vi "PID_RT.vi"() -> ()   [LabVIEW 2017]
uses:
  <vilib>/myRIO/Instrument Drivers/Onboard IO/AO/typedefs/AO Reference.ctl
  <vilib>/myRIO/Common/Instrument Driver Framework/Utilities/typedefs/myRIO Generic Hardware Reference.ctl
  <vilib>/myRIO/Common/Instrument Driver Framework/Utilities/typedefs/Hardware Version Enum.ctl
  <vilib>/myRIO/Common/Instrument Driver Framework/Utilities/typedefs/myRIO v1.0 Reference.ctl
  <vilib>/myRIO/Common/Instrument Driver Framework/Utilities/typedefs/Generic FPGA Reference.ctl
  <vilib>/myRIO/Common/Instrument Driver Framework/myRIO v1.0/AO/typedefs/AO Channels List.ctl
  <vilib>/myRIO/Common/Instrument Driver Framework/myRIO v1.0/AO/typedefs/AO Channels Enum.ctl
  <vilib>/myRIO/Common/Instrument Driver Framework/Utilities/typedefs/Analog Scaling Constants List.ctl
  <vilib>/myRIO/Common/Instrument Driver Framework/Utilities/typedefs/Analog Scaling Constants.ctl
  <vilib>/userdefined/High Color/nirio_resource_hc.ctl
  <vilib>/Platform/TimedLoop/XDataNode/timing_clust.ctl
  <vilib>/Platform/TimedLoop/XDataNode/nitl_modes.ctl
  <vilib>/Platform/TimedLoop/XDataNode/wakeup.ctl
  <vilib>/myRIO/Common/Instrument Driver Framework/Utilities/vis/Is FPGA Ref Available.vi
  <vilib>/myRIO/Common/Instrument Driver Framework/myRIO v1.0/AO/vis/myRIO v1.1 Open AO.vi
  <vilib>/myRIO/Instrument Drivers/Onboard IO/AO/vis/Write.vi
  <vilib>/myRIO/Common/Instrument Driver Framework/Utilities/vis/Validate Channels.vi
  <vilib>/myRIO/Common/Instrument Driver Framework/myRIO v1.0/AO/vis/myRIO v1.0 Reserve AO.vi
  <vilib>/myRIO/Common/Instrument Driver Framework/myRIO v1.0/AO/vis/myRIO v1.0 Build MUX Configuration AO.vi
  <vilib>/myRIO/Common/Instrument Driver Framework/myRIO v1.0/Resource Manager/vis/myRIO v1.0 Reserve Channel List.vi
  <vilib>/myRIO/Common/Instrument Driver Framework/myRIO v1.0/Resource Manager/vis/myRIO v1.0 Reserve Channel.vi
  <vilib>/myRIO/Common/Instrument Driver Framework/myRIO v1.0/Resource Manager/vis/myRIO v1.0 Unreserve Channel.vi
  <vilib>/myRIO/Common/Instrument Driver Framework/myRIO v1.0/Resource Manager/vis/myRIO v1.0 Build Mutex Name.vi
  <vilib>/Utility/VariantDataType/GetNumericInfo.vi
  <vilib>/Utility/error.llb/Error Cluster From Error Code.vi
  <vilib>/myRIO/Common/Instrument Driver Framework/myRIO v1.0/myRIO v1.1 Open.vi
  <vilib>/myRIO/Common/Instrument Driver Framework/myRIO v1.0/AO/vis/myRIO v1.0 Get Scaling Constants AO.vi
  <vilib>/myRIO/Common/Instrument Driver Framework/Utilities/vis/IO Manager.vi
  <vilib>/myRIO/Common/Instrument Driver Framework/Utilities/vis/Configuration Manager.vi
  <vilib>/myRIO/Common/Instrument Driver Framework/myRIO v1.0/myRIO v1.0 Close.vi
  <vilib>/myRIO/Common/Instrument Driver Framework/myRIO v1.0/AO/vis/myRIO v1.0 Write AO.vi
  <vilib>/addons/control/pid/pid.llb/PID (DBL).vi
  <vilib>/myRIO/Express VI/Onboard IO/AO/AO Express VI.xnode
  <vilib>/myRIO/Instrument Drivers/Onboard IO/AO/vis/myRIO AO Open.xnode
  <vilib>/platform/TimedLoop/XDataNode/XDataNode.xnode
  <vilib>/addons/control/pid/NI_PID_pid.lvlib
  <vilib>/myRIO/Instrument Drivers/Onboard IO/AO/AO.lvlib
  <vilib>/Platform/TimedLoop/XDataNode/XDNodeRunTimeDep.lvlib
panel:
  out "Yel":bool
  out "Red":bool
  out "Grn":bool
  out "Speeding Up?":bool
  out "Velocity":dbl(graph)
  in  "stop":bool
  out "error out":errorcluster
  out "process variable":dbl
  out "Setpoint":dbl
  out "Analog Output":dbl(graph)=3.193359702
  out "output":dbl format="%.2f"
  out "Theta":cluster{"setpoint":dbl, dbl}(graph)={"setpoint"=303.908879655711, 0.0}
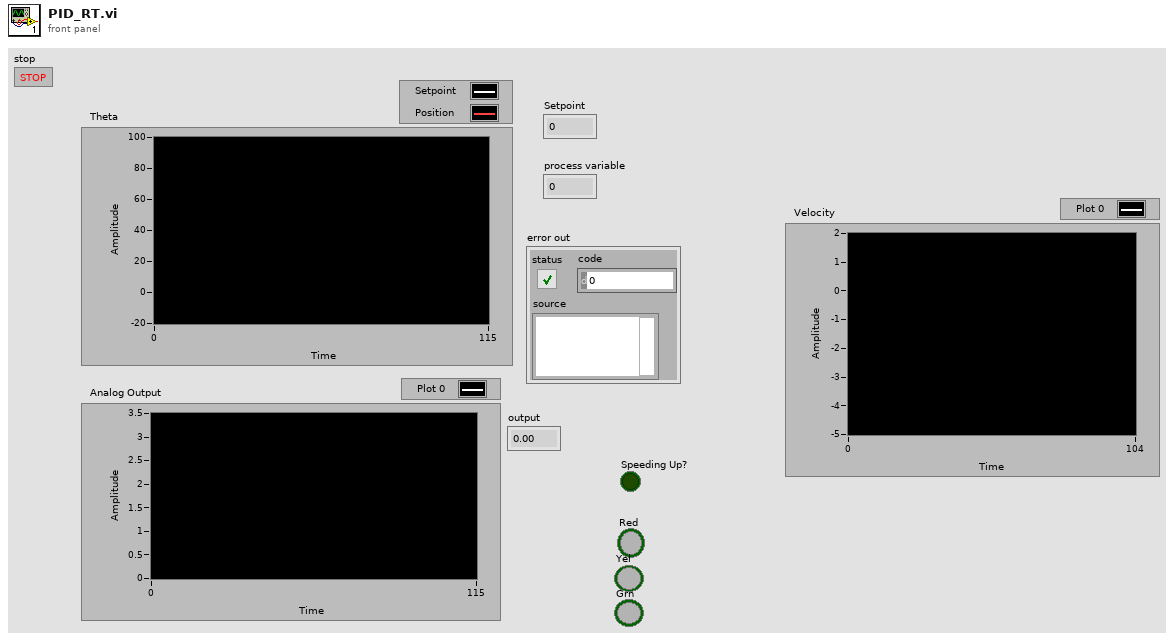
[diagram p1: front panel]
types:
  T1 = typedef "AO.lvlib/AO Reference.ctl" = cluster{"myRIO Reference":T2, "AO Channel List":T6, "AO Scaling Constant List":T8}
  T2 = typedef "myRIO Generic Hardware Reference.ctl" = cluster{"myRIO Model":T3, "myRIO Hardware Reference":T4}
  T3 = typedef "Hardware Version Enum.ctl" = enum16{"Unknown", "myRIO-1900", "myRIO-1950", "roboRIO", "NI ELVIS RIO CM"}
  T4 = typedef "myRIO v1.0 Reference.ctl" = cluster{"Generic FPGA Reference":T5, "Allow multiple opens":bool}
  T5 = typedef "Generic FPGA Reference.ctl" = refnum<k20>
  T6 = typedef "AO Channels List.ctl" = T7[]
  T7 = typedef "AO Channels Enum.ctl" = enum16{"Not Connected", "AudioOut/Left", "AudioOut/Right", "C/AO0", "C/AO1", "A/AO0", "A/AO1", "B/AO0", "B/AO1"}
  T8 = typedef "Analog Scaling Constants List.ctl" = T9[]
  T9 = typedef "Analog Scaling Constants.ctl" = cluster{"LSB Weight (Volts)":dbl, "Offset (Volts)":dbl, "Signed?":bool}
  T10 = typedef "nirio_resource_hc.ctl" = tag
  T11 = typedef "XDNodeRunTimeDep.lvlib/timing_clust.ctl" = cluster{"Expected End [f-1]":u64, "Actual End [f-1]":u64, "Finished Late? [f-1]":bool, "Expected End [i-1]":u64, "Actual End [i-1]":u64, "Finished Late? [i-1]":bool, "Expected Start [i]":u64, "Actual Start [i]":u64, "Expected Start [f]":u64, "Actual Start [f]":u64, "Source Name":string, "Structure Name":string, "Period":i64, "Deadline":i64, "Offset":i64, "Start":i64, "Priority":i32, "Timeout":i32, "Mode":T12, "Wakeup Reason":T13, "Error":errorcluster, "Source Type":string, "Secondary Source Type":string, "Global End Time":u64, "Global Start Time":u64, "Frame Duration":u64, "Iteration Duration":u64, "Assigned CPU":i32, "I/O Scan Engine Mode":u32}
  T12 = typedef "XDNodeRunTimeDep.lvlib/nitl_modes.ctl" = enum32{"No Change", "Process missed periods, maintain original phase", "Discard missed periods, maintain original phase", "Process missed periods, ignore original phase", "Discard missed periods, ignore original phase"}
  T13 = typedef "XDNodeRunTimeDep.lvlib/wakeup.ctl" = enum32{"Normal", "Aborted", "Asynchronous wakeup", "Timing source error", "Timed loop error", "Timeout"}
  T14 = cluster{"proportional gain (Kc)":dbl, "integral time (Ti, min)":dbl, "derivative time (Td, min)":dbl}
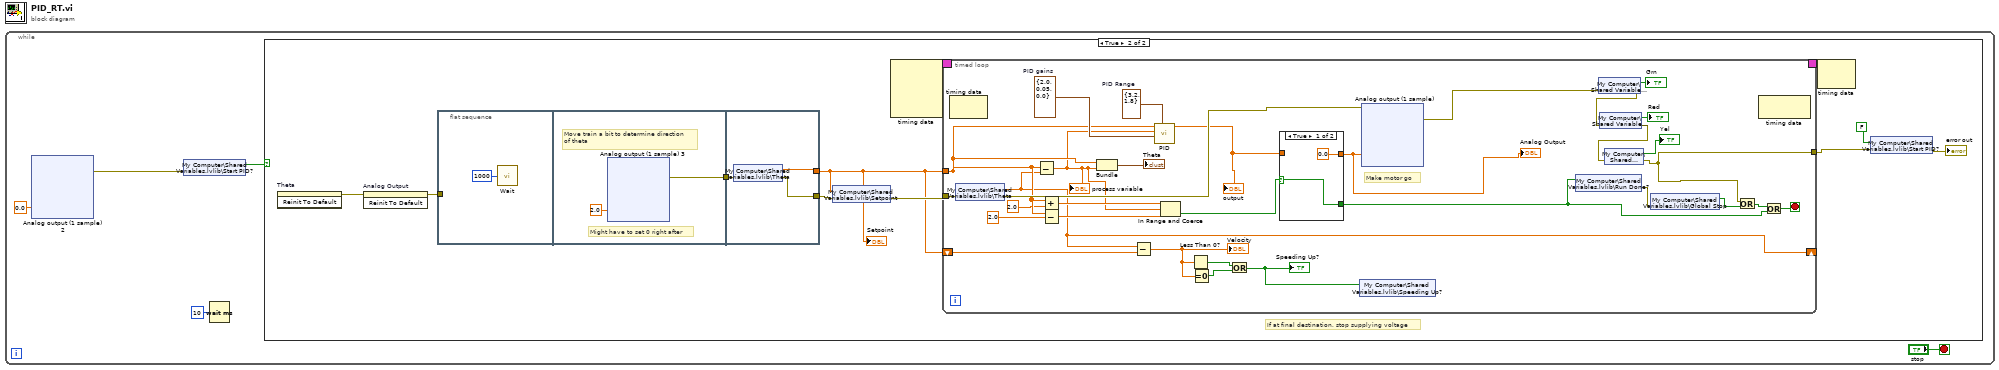
[diagram p0: block diagram]
diagram:
  n1 = while {
    stop <- "stop" stop-if-true
    n2 = xnode "Analog output (1 sample) 2"("C/AO0 (AO0)"=0.0) -> ("error out"=w1:errorcluster)  [unwired: 1 in]
    n3 = shared-variable "My Computer\\Shared Variables.lvlib\\Start PID?"(error in=w1) -> (w4:bool)  [unwired: 1 out]
    n4 = Wait (ms)(milliseconds to wait=u32 10) -> ()  [unwired: 1 out]
    n5 = case shown="True" w4 {
      frame False {
      }
      frame True {
        # "If at final destination, stop supplying voltage"
        n6 = invoke on="Theta" class="WFChart (strict)" method="Reinit To Default"() -> (error out=w50:errorcluster)  [unwired: 3 in, 2 out]
        n7 = invoke on="Analog Output" class="WFChart (strict)" method="Reinit To Default"(error in=w50) -> (error out=w49:errorcluster)  [unwired: 2 in, 2 out]
        n8 = flat-sequence {
          tunnel: w49 -> [_]
          tunnel: [w55] -> w51
          tunnel: [w96] -> w43
          tunnel: [w95] -> w48
          tunnel: w51 -> [w94]
          frame #0 {
            n9 = call "Wait"("Count(mSec)"=u32 1000) -> ()  [unwired: 1 out]
          }
          frame #1 {
            # "Might have to set 0 right after"
            # "Move train a bit to determine direction\nof theta"
            n10 = xnode "Analog output (1 sample) 3"("C/AO0 (AO0)"=2.0) -> ("error out"=w55:errorcluster)  [unwired: 1 in]
          }
          frame #2 {
            n11 = shared-variable "My Computer\\Shared Variables.lvlib\\Theta"(error in=w94) -> (w96:dbl, error out=w95:errorcluster)
          }
        }
        n12 = shared-variable "My Computer\\Shared Variables.lvlib\\Setpoint"(w43, error in=w48) -> (error out=w47:errorcluster)
        n13 = node-c288() -> (w53:T11)  [unwired: 4 in]
        n14 = timed-loop {
          timing: w53 -> [_]
          timing-out: [_] -> w52
          tunnel: w43 -> [w123]
          tunnel: w47 -> [w125]
          tunnel: [w97] -> w46
          shift-right: [w108] -> _
          shift-left: w43 -> [w109]
          stop <- w114 stop-if-true
          w127 = T14 {"proportional gain (Kc)"=2.0, "integral time (Ti, min)"=0.05, "derivative time (Td, min)"=0.0}  # PID gains
          w128 = cluster{"output high":dbl, "output low":dbl} {"output high"=3.2, "output low"=1.8}  # PID Range
          # "Make motor go"
          n15 = node-c288() -> ()  [unwired: 1 in, 1 out]
          n16 = shared-variable "My Computer\\Shared Variables.lvlib\\Theta"(error in=w125) -> (w108:dbl, error out=w124:errorcluster)
          n17 = Subtract(x=w123, y=w108) -> (x-y=w110:dbl)
          "process variable" <- w110
          n18 = Add(x=w123, y=2.0) -> (x+y=w120:dbl)
          n19 = Subtract(x=w123, y=2.0) -> (x-y=w119:dbl)
          n20 = Bundle("Double"=w123, w110) -> (→"Theta":cluster{"Double":dbl, dbl})  [unwired: 1 in]
          n21 = Subtract(x=w108, y=w109) -> (x-y=w106:dbl)
          "Velocity" <- w106
          n22 = call-poly <vilib>:"PID.vi"("output range"=w128, "PID gains"=w127, "process variable"=w110, "setpoint"=w123) -> ("output"=w117:dbl)  [unwired: 6 in, 1 out]
          "output" <- w117
          n23 = In Range and Coerce(upper limit=w120, x=w110, lower limit=w119) -> (In Range?=w118:bool)  [unwired: 1 out]
          n24 = Less Than 0?(x=w106) -> (x < 0?=w107:bool)
          n25 = Equal To 0?(x=w106) -> (x = 0?=w105:bool)
          n26 = Or(x=w107, y=w105) -> (x .or. y?=w104:bool)
          "Speeding Up?" <- w104
          n27 = case shown="True" w118 {
            selector: w118 -> [w129 w131]
            tunnel: [0.0 ("output") w132] -> w116
            tunnel: w117 -> [_ w132]
            tunnel: [w129 w131] -> w112
            frame True {
            }
            frame False {
            }
          }
          "Analog Output" <- w116
          n28 = shared-variable "My Computer\\Shared Variables.lvlib\\Speeding Up?"(w104) -> ()  [unwired: 1 in, 1 out]
          n29 = xnode "Analog output (1 sample)"("C/AO0 (AO0)"=w116, "error in (no error)"=w124) -> ("error out"=w103:errorcluster)
          n30 = shared-variable "My Computer\\Shared Variables.lvlib\\Run Done?"(w112) -> (error out=w111:errorcluster)  [unwired: 1 in]
          n31 = shared-variable "My Computer\\Shared Variables.lvlib\\Grn"(error in=w103) -> (→"Grn":bool, error out=w102:errorcluster)
          n32 = shared-variable "My Computer\\Shared Variables.lvlib\\Red"(error in=w102) -> (→"Red":bool, error out=w101:errorcluster)
          n33 = shared-variable "My Computer\\Shared Variables.lvlib\\Yel"(error in=w101) -> (→"Yel":bool, error out=w97:errorcluster)
          n34 = shared-variable "My Computer\\Shared Variables.lvlib\\Global Stop"(error in=w111) -> (w115:bool)  [unwired: 1 out]
          n35 = Or(x=w97, y=w115) -> (x .or. y?=w113:bool)
          n36 = node-c288() -> ()  [unwired: 1 in, 1 out]
          n37 = Or(x=w113, y=w112) -> (x .or. y?=w114:bool)
        }
        n38 = node-c288(w52) -> ()  [unwired: 1 out]
        n39 = shared-variable "My Computer\\Shared Variables.lvlib\\Start PID?"(FALSE ("Start PID?"), error in=w46) -> (error out=→"error out":errorcluster)
        "Setpoint" <- w43
      }
    }
  }
